vi "Script Express VI.vi"(4 "Variant":string, 5 "Special Terminals":T1={"Action"=-1, "Init"=-1, "Tag"=-1, "State in"=-1, "State out"=-1, "Error"=-1}, 6 "Worker":string, 7 "Flattened Icon":T2, 8 "Terminal Configs":T3[](array[typedef]), 9 "VI":refnum<vi>, 10 "ParentVI":refnum<vi>, 11 "subVI":refnum<vi>) -> (0 "error out":errorcluster)   [LabVIEW 2020, in "FlexBlocks.lvlib"]
uses:
  FlexBlocks.lvlib
  Terminal Config.ctl
  Type Descriptor.ctl
  Terminal Direction.ctl
  Value Mode.ctl
  Special Terminal.ctl
  Terminal Mode.ctl
  <vilib>/picture/picture.llb/imagedata.ctl
  Special Terminal Indices.ctl
  Scripting Refs.ctl
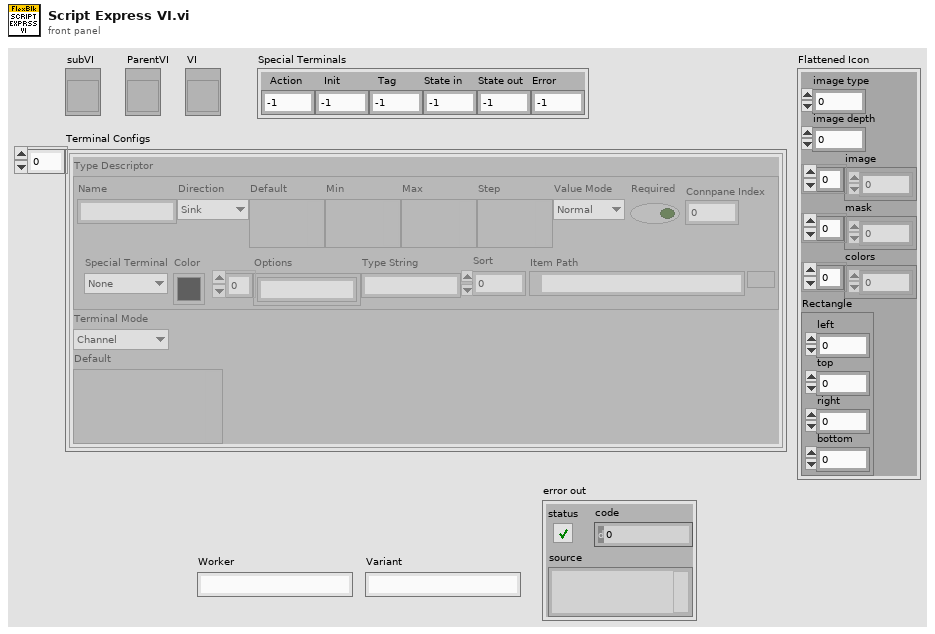
[diagram p1: front panel]
types:
  T1 = typedef "FlexBlocks.lvlib/Special Terminal Indices.ctl" = cluster{"Action":i32, "Init":i32, "Tag":i32, "State in":i32, "State out":i32, "Error":i32}
  T2 = typedef "imagedata.ctl" = cluster{"image type":i32, "image depth":i32, "image":u8[], "mask":u8[], "colors":u32[], "Rectangle":cluster{"left":i16, "top":i16, "right":i16, "bottom":i16}}
  T3 = typedef "FlexBlocks.lvlib/Terminal Config.ctl" = cluster{"Type Descriptor":T4, "Terminal Mode":T8, "Default":variant}
  T4 = typedef "FlexBlocks.lvlib/Type Descriptor.ctl" = cluster{"Name":string, "Direction":T5, "Default":variant, "Min":variant, "Max":variant, "Step":variant, "Value Mode":T6, "Required":bool, "Connpane Index":i32, "Special Terminal":T7, "Color":u32, "Options":string[], "Type String":string, "Sort":i32, "Item Path":path}
  T5 = typedef "FlexBlocks.lvlib/Terminal Direction.ctl" = enum16{"Sink", "Source"}
  T6 = typedef "FlexBlocks.lvlib/Value Mode.ctl" = enum16{"Normal", "Range", "Select"}
  T7 = typedef "FlexBlocks.lvlib/Special Terminal.ctl" = enum16{"None", "Action", "Init", "Tag", "State in", "State out", "Error"}
  T8 = typedef "FlexBlocks.lvlib/Terminal Mode.ctl" = enum16{"Channel", "Config", "Value", "Control Ref"}
  T9 = typedef "FlexBlocks.lvlib/Scripting Refs.ctl" = cluster{"VI":refnum<vi>, "subVI":refnum<vi>, "Work SVR":refnum<vi>, "SVR DDS":refnum<vi>, "CBR DDS":refnum<vi>, "Init DDS":refnum<vi>, "Tag DDS":refnum<vi>, "Terminals":refnum<vi>[], "First Init":refnum<vi>, "First Work":refnum<vi>, "First Source":refnum<vi>, "Input CS":refnum<vi>, "Input Stops":refnum<vi>, "Status Stops":refnum<vi>, "Tag BBN":refnum<vi>, "Init Term":refnum<vi>, "Tag Term":refnum<vi>, "State Term":refnum<vi>, "Output CS":refnum<vi>, "Init BBN":refnum<vi>, "CBR":refnum<vi>, "Work CS":refnum<vi>, "Worker Error":refnum<vi>}
  T10 = typedef "FlexBlocks.lvlib/Grouped Terminals.ctl" = cluster{"Init":T11, "Work":T11, "Source":T11}
  T11 = typedef "FlexBlocks.lvlib/Terminal Group.ctl" = cluster{"Terminals":refnum<vi>[], "Types":T3[]}
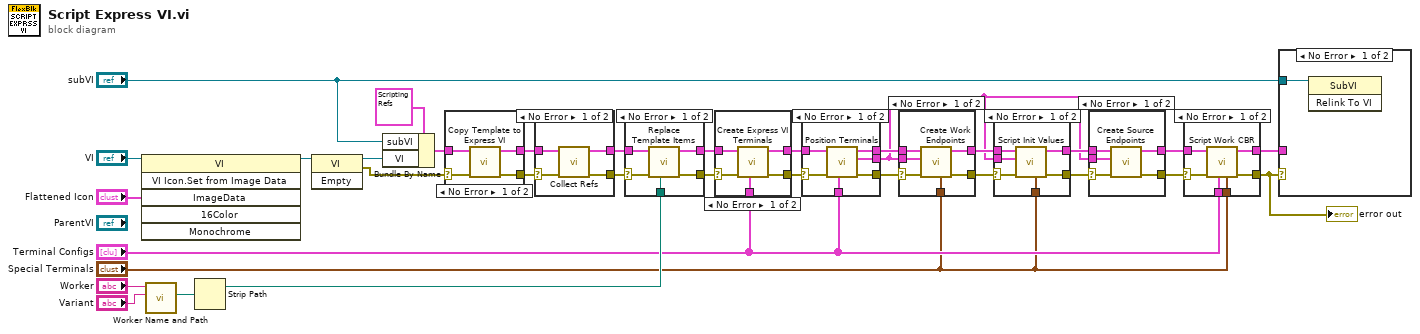
[diagram p0: block diagram]
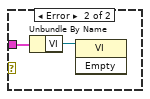
[diagram p11: hidden frame]
diagram:
  n1 = invoke class="VI" method="VI Icon.Set from Image Data"(reference="VI", "ImageData"="Flattened Icon") -> (reference out=w31:refnum<vi>)  [unwired: 4 in, 5 out]
  n2 = call "Worker Name and Path.vi"("Variant"="Variant", "Worker"="Worker") -> ("lvlib Path"=w27:path)  [unwired: 6 in, 3 out]
  n3 = Strip Path(path=w27) -> (stripped path=w21:path)  [unwired: 1 out]
  n4 = invoke class="VI" method="Empty"(reference=w31) -> (reference out=w19:refnum<vi>, error out=w25:errorcluster)  [unwired: 2 in, 1 out]
  n5 = Bundle By Name(cluster=T9 {"VI"=refnum, "subVI"=refnum, "Work SVR"=refnum, "SVR DDS"=refnum, "CBR DDS"=refnum, "Init DDS"=refnum, "Tag DDS"=refnum, "Terminals"=[], "First Init"=refnum, "First Work"=refnum, "First Source"=refnum, "Input CS"=refnum, "Input Stops"=refnum, "Status Stops"=refnum, "Tag BBN"=refnum, "Init Term"=refnum, "Tag Term"=refnum, "State Term"=refnum, "Output CS"=refnum, "Init BBN"=refnum, "CBR"=refnum, "Work CS"=refnum, "Worker Error"=refnum} ("Refs in"), "subVI"="subVI", "VI"=w19) -> (w18:T9)
  n6 = case shown="No Error" w25 {
    selector: w25 -> [w37 w39]
    tunnel: [w36 w39] -> w24
    tunnel: w18 -> [w35 w38]
    tunnel: [w34 w38] -> w17
    frame No Error {
      n7 = call "Copy Template to Express VI.vi"("error in (no error)"=w37, "Refs in"=w35) -> ("error out"=w36:errorcluster, "Refs"=w34:T9)  [unwired: 8 in]
    }
    frame Error {
    }
  }
  n8 = case shown="No Error" w24 {
    selector: w24 -> [w43 w45]
    tunnel: [w42 w45] -> w22
    tunnel: w17 -> [w41 w44]
    tunnel: [w40 w44] -> w16
    frame No Error {
      n9 = call "Collect Refs.vi"("error in (no error)"=w43, "Refs in"=w41) -> ("error out"=w42:errorcluster, "Refs"=w40:T9)  [unwired: 8 in]
    }
    frame Error {
    }
  }
  n10 = case shown="No Error" w22 {
    selector: w22 -> [w50 w52]
    tunnel: [w49 w52] -> w20
    tunnel: w21 -> [w48 _]
    tunnel: w16 -> [w47 w51]
    tunnel: [w46 w51] -> w15
    frame No Error {
      n11 = call "Replace Template Items.vi"("Worker Folder"=w48, "error in (no error)"=w50, "Refs in"=w47) -> ("error out"=w49:errorcluster, "Refs"=w46:T9)  [unwired: 7 in]
    }
    frame Error {
    }
  }
  n12 = case shown="No Error" w20 {
    selector: w20 -> [w55 w59]
    tunnel: "Terminal Configs" -> [w57 _]
    tunnel: [w56 w59] -> w26
    tunnel: w15 -> [w54 w58]
    tunnel: [w53 w58] -> w14
    frame No Error {
      n13 = call "Create Express VI Terminals.vi"("Terminal Configs"=w57, "error in (no error)"=w55, "Refs in"=w54) -> ("error out"=w56:errorcluster, "Refs"=w53:T9)  [unwired: 7 in]
    }
    frame Error {
    }
  }
  n14 = case shown="No Error" w26 {
    selector: w26 -> [w65 w67]
    tunnel: [w64 w67] -> w30
    tunnel: "Terminal Configs" -> [w63 _]
    tunnel: [w62 _] -> w3
    tunnel: w14 -> [w61 w66]
    tunnel: [w60 w66] -> w13
    frame No Error {
      n15 = call "Position Terminals.vi"("Terminal Configs"=w63, "error in (no error)"=w65, "Refs in"=w61) -> ("error out"=w64:errorcluster, "Grouped Terminals"=w62:T10, "Refs"=w60:T9)  [unwired: 6 in]
    }
    frame Error {
    }
  }
  n16 = case shown="No Error" w30 {
    selector: w30 -> [w73 w75]
    tunnel: [w72 w75] -> w11
    tunnel: w3 -> [w71 _]
    tunnel: w13 -> [w70 w74]
    tunnel: [w69 w74] -> w10
    tunnel: "Special Terminals" -> [w68 _]
    frame No Error {
      n17 = call "Create Work Endpoints.vi"("Special Terminals"=w68, "error in (no error)"=w73, "Grouped Terminals"=w71, "Refs in"=w70) -> ("error out"=w72:errorcluster, "Refs"=w69:T9)  [unwired: 6 in]
    }
    frame Error {
    }
  }
  n18 = case shown="No Error" w11 {
    selector: w11 -> [w81 w83]
    tunnel: [w80 w83] -> w8
    tunnel: w3 -> [w79 _]
    tunnel: w10 -> [w78 w82]
    tunnel: [w77 w82] -> w9
    tunnel: "Special Terminals" -> [w76 _]
    frame No Error {
      n19 = call "Script Init Values.vi"("Special Terminals"=w76, "error in (no error)"=w81, "Grouped Terminals"=w79, "Refs in"=w78) -> ("error out"=w80:errorcluster, "Refs"=w77:T9)  [unwired: 6 in]
    }
    frame Error {
    }
  }
  n20 = case shown="No Error" w8 {
    selector: w8 -> [w88 w90]
    tunnel: [w87 w90] -> w6
    tunnel: w3 -> [w86 _]
    tunnel: w9 -> [w85 w89]
    tunnel: [w84 w89] -> w7
    frame No Error {
      n21 = call "Create Source Endpoints.vi"("error in (no error)"=w88, "Grouped Terminals"=w86, "Refs in"=w85) -> ("error out"=w87:errorcluster, "Refs"=w84:T9)  [unwired: 7 in]
    }
    frame Error {
    }
  }
  n22 = case shown="No Error" w6 {
    selector: w6 -> [w95 w98]
    tunnel: [w94 w98] -> w5
    tunnel: w7 -> [w96 w97]
    tunnel: [w93 w97] -> w4
    tunnel: "Terminal Configs" -> [w92 _]
    tunnel: "Special Terminals" -> [w91 _]
    frame No Error {
      n23 = call "Script Work CBR.vi"("Special Terminals"=w91, "Terminal Configs"=w92, "error in (no error)"=w95, "Refs in"=w96) -> ("error out"=w94:errorcluster, "Refs"=w93:T9)  [unwired: 6 in]
    }
    frame Error {
    }
  }
  "error out" <- w5
  n24 = case shown="No Error" w5 {
    tunnel: "subVI" -> [w99 _]
    tunnel: w4 -> [_ w101]
    frame No Error {
      n25 = invoke class="SubVI" method="Relink To VI"(reference=w99) -> ()  [unwired: 2 in, 3 out]
    }
    frame Error {
      n26 = Unbundle By Name(w101) -> ("VI"=w100:refnum<vi>)
      n27 = invoke class="VI" method="Empty"(reference=w100) -> ()  [unwired: 2 in, 3 out]
    }
  }
